vi "Read activeBridge.vi"(11 "TestMonitor in":refnum<class "TestMonitor.lvclass">) -> (2 "activeBridge":u32 min=1, 3 "TestMonitor out":refnum<class "TestMonitor.lvclass">)   [LabVIEW 2013, in "TestMonitor.lvclass"]
uses:
  TestMonitor.lvclass
  TestMonitor.lvclass/TestMonitor.ctl
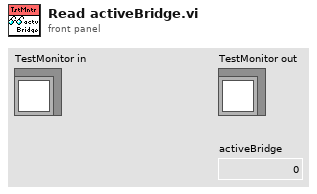
[diagram p1: front panel]
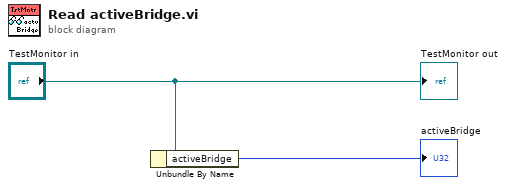
[diagram p0: block diagram]
diagram:
  n1 = Unbundle By Name("TestMonitor in") -> ("activeBridge"=→"activeBridge":u32)
  "TestMonitor out" <- "TestMonitor in"
